vi "reverse_tachometer_counter.vi"() -> ()   [LabVIEW 2014]
uses:
  <vilib>/Analysis/baseanly.llb/Mean (DBL).vi
  <vilib>/DAQmx/create/channels.llb/DAQmx Create Channel (CI-Pulse Width).vi
  <vilib>/DAQmx/read.llb/DAQmx Read (Counter 1D DBL 1Chan NSamp).vi
  <vilib>/Analysis/NI_AALBase.lvlib
panel:
  out "XY Graph":cluster{"X":dbl, "Y":dbl}[](graph)
  in  "Save file":path
  out "Voltage [V]":dbl format="%#_2p"
  in  "calibration file":path=path "C:/Users/jensv_000/LabVIEW/reverse_tachometer_counter/Docs/calibration/2015-07/calibration.csv"
  in  "Voltage Divide Factor":dbl=1.0
  out "Pulse Width [s]":dbl format="%#_3p"
  in  "Save & Close":bool
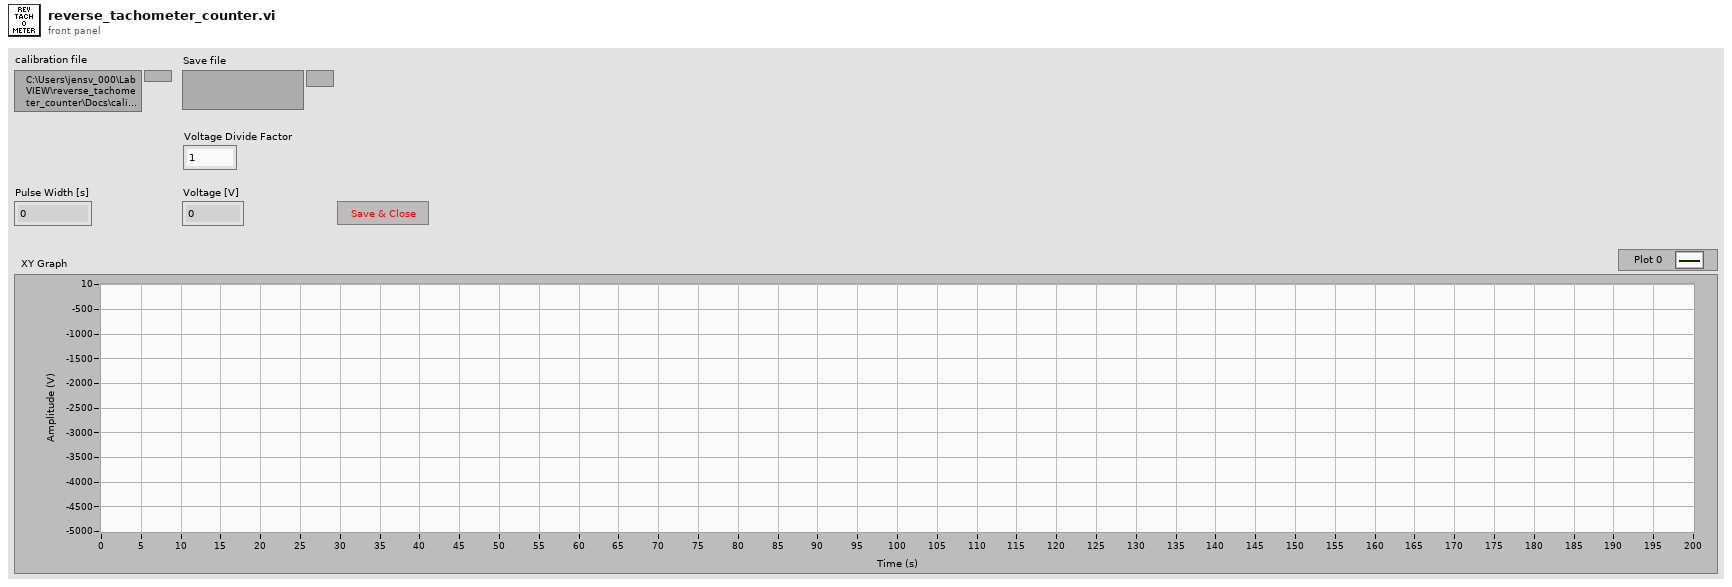
[diagram p1: front panel]
types:
  T1 = enum16{"open", "replace", "create", "open or create", "replace or create", "replace or create with confirmation"}
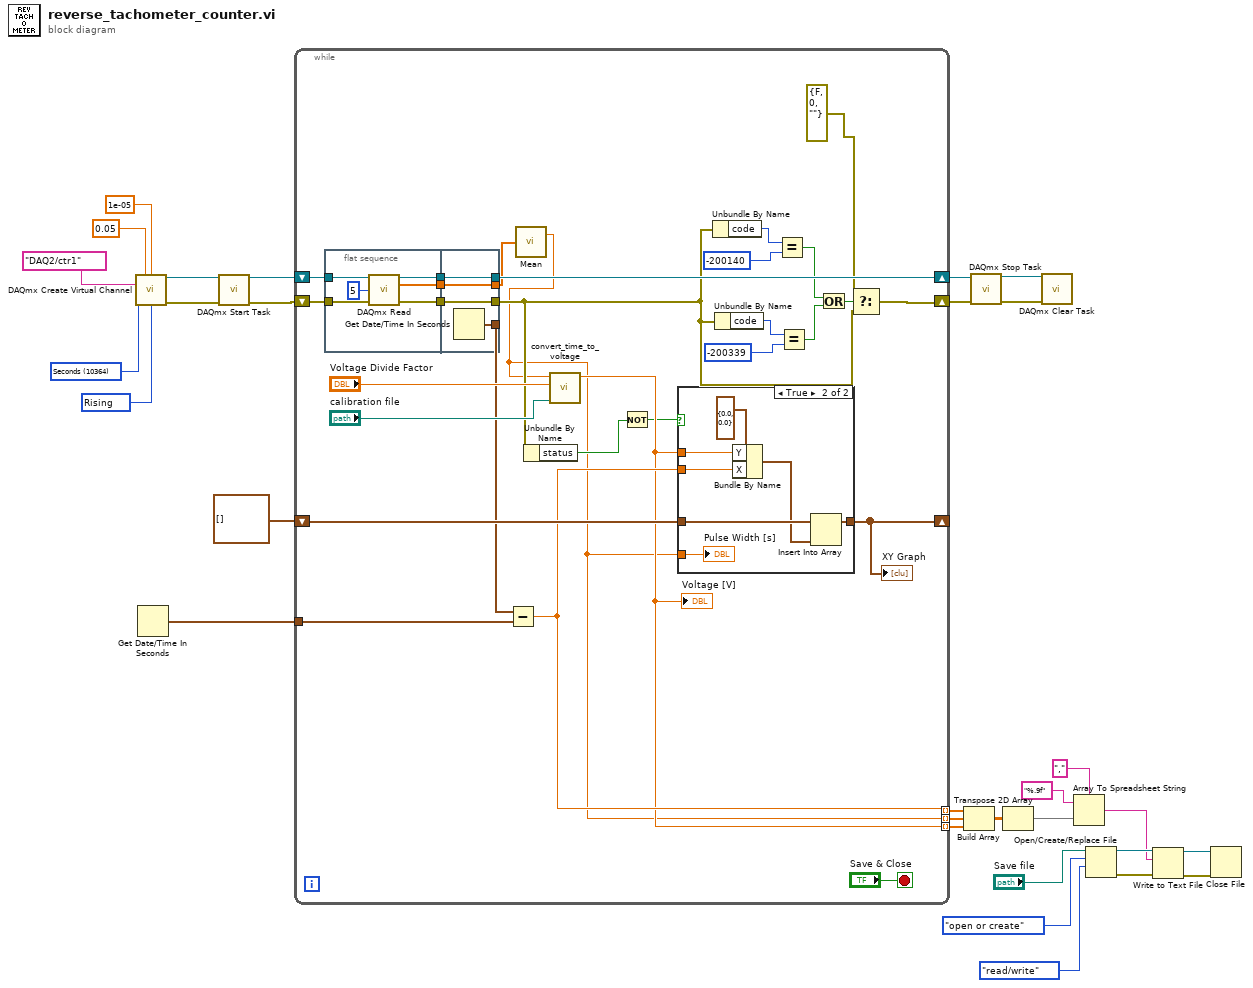
[diagram p0: block diagram]
diagram:
  w18 = 10280 items=["Rising"=10280, "Falling"=10171] ("starting edge")
  w19 = 10364 items=["Seconds"=10364, "Ticks"=10304, "From Custom Scale"=10065] ("units")
  n1 = call-poly <vilib>:"DAQmx Create Virtual Channel.vi"("maximum value"=0.05, "minimum value"=1e-05, "counter"=tag "DAQ2/ctr1", "units"=w19, "starting edge"=w18) -> ("task out"=w25:refnum<k21>, "error out"=w24:errorcluster)  [unwired: 9 in]
  n2 = Get Date/Time In Seconds() -> (seconds since 1Jan1904=w4:timestamp)
  n3 = call <vilib>:"DAQmx Start Task.vi"("task/channels in"=w25, "error in"=w24) -> ("task out"=w22:refnum<k21>, "error out"=w23:errorcluster)  [unwired: 12 in]
  n4 = while {
    shift-right: [w53] -> w26
    shift-left: w23 -> [w58]
    shift-right: [w59] -> w27
    shift-left: w22 -> [w57]
    shift-right: [w44] -> _
    shift-left: cluster{"X":dbl, "Y":dbl}[] [] ("XY Graph") -> [w49]
    tunnel: [w45] -> w10 mode=indexing
    tunnel: [w32] -> w9 mode=indexing
    tunnel: [w41] -> w8 mode=indexing
    tunnel: w4 -> [w42]
    stop <- "Save & Close" stop-if-true
    n5 = flat-sequence {
      tunnel: w58 -> [w72]
      tunnel: w57 -> [w71]
      tunnel: [w73] -> w48
      tunnel: [w70] -> w47
      tunnel: [w69] -> w46
      tunnel: [w75] -> w33
      tunnel: [w76] -> w35
      tunnel: [w77] -> w59
      tunnel: w48 -> [w77]
      tunnel: w47 -> [w76]
      tunnel: w46 -> [w75]
      tunnel: [w74] -> w43
      frame #0 {
        n6 = call-poly <vilib>:"DAQmx Read.vi"("task/channels in"=w71, "number of samples per channel"=5, "error in"=w72) -> ("task out"=w73:refnum<k21>, "data"=w69:dbl[], "error out"=w70:errorcluster)  [unwired: 10 in]
      }
      frame #1 {
        n7 = Get Date/Time In Seconds() -> (seconds since 1Jan1904=w74:timestamp)
      }
    }
    n8 = Subtract(x=w43, y=w42) -> (x-y=w45:dbl)
    n9 = call-poly <vilib>:"Mean.vi"("X"=w33) -> ("mean"=w32:dbl)  [unwired: 1 out]
    n10 = Unbundle By Name(w35) -> ("status"=w34:bool)
    n11 = call "convert_time_to_voltage.vi"("calibration file"="calibration file", "Voltage Divide Factor"="Voltage Divide Factor", "measurement"=w32) -> ("Voltage"=w41:dbl)  [unwired: 8 in]
    "Voltage [V]" <- w41
    n12 = Not(x=w34) -> (.not. x?=w31:bool)
    n13 = case shown="True" w31 {
      tunnel: w49 -> [w60 w67]
      tunnel: w45 -> [_ w65]
      tunnel: [w60 w63] -> w44
      tunnel: w41 -> [_ w62]
      tunnel: w32 -> [_ w61]
      frame False {
      }
      frame True {
        n14 = Bundle By Name(cluster=cluster{"X":dbl, "Y":dbl} {"X"=0.0, "Y"=0.0}, "Y"=w62, "X"=w65) -> (w64:cluster{"X":dbl, "Y":dbl})
        n15 = Insert Into Array(array=w67, new element=w64) -> (w63:cluster{"X":dbl, "Y":dbl}[])  [unwired: 1 in]
        "Pulse Width [s]" <- w61
      }
    }
    "XY Graph" <- w44
    n16 = Unbundle By Name(w35) -> ("code"=w40:i32)
    n17 = Unbundle By Name(w35) -> ("code"=w55:i32)
    n18 = Equal?(x=w40, y=-200140) -> (x = y?=w37:bool)
    n19 = Equal?(x=w55, y=-200339) -> (x = y?=w36:bool)
    n20 = Or(x=w37, y=w36) -> (x .or. y?=w38:bool)
    n21 = Select(t=errorcluster {"status"=FALSE, "code"=0, "source"=""} ("s? t:f"), s=w38, f=w35) -> (s? t:f=w53:errorcluster)
  }
  n22 = Build Array(w10, w9, w8) -> (w2:dbl[][])
  n23 = call <vilib>:"DAQmx Stop Task.vi"("task/channels in"=w27, "error in"=w26) -> ("task out"=w21:refnum<k21>, "error out"=w20:errorcluster)  [unwired: 12 in]
  n24 = Transpose 2D Array(2D array=w2) -> (transposed array=w1:dbl[][])
  n25 = call <vilib>:"DAQmx Clear Task.vi"("task in"=w21, "error in"=w20) -> ()  [unwired: 13 in, 1 out]
  n26 = Array To Spreadsheet String(delimiter (Tab)=",", array=w1, 3:"%.9f" ("format string")) -> (spreadsheet string=w7:string)
  n27 = Open/Create/Replace File(file path (use dialog)="Save file", operation (0:open)=T1."open or create", access (0:read/write)=enum16{"read/write", "read-only", "write-only"}."read/write") -> (refnum out=w17:refnum<file>, error out=w16:errorcluster)  [unwired: 3 in, 1 out]
  n28 = Write to Text File(file (use dialog)=w17, text=w7, error in=w16) -> (refnum out=w15:refnum<file>, error out=w14:errorcluster)  [unwired: 1 in, 1 out]
  n29 = Close File(refnum=w15, error in=w14) -> ()  [unwired: 2 out]
